vi "QuickSort(Unsigned Byte).vi"(11 "Array In":u8[](array[numeric])) -> (1 "Indices Out":i32[](array[numeric]), 3 "Array Out":u8[](array[numeric]))   [LabVIEW 2015, in "Sorting.lvlib"]
uses:
  Sorting.lvlib
  QSHelper Instances/QSHelper(Unsigned Byte).vi
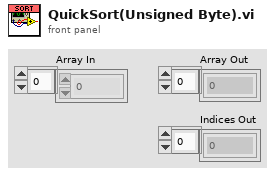
[diagram p1: front panel]
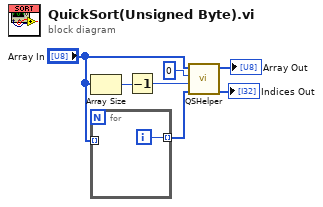
[diagram p0: block diagram]
diagram:
  n1 = Array Size(array="Array In") -> (size(s)=w6:i32)
  n2 = for {
    tunnel: "Array In" -> [_] mode=indexing
    tunnel: [w8] -> w2 mode=indexing
    i -> [w8]
  }
  n3 = Decrement(x=w6) -> (x-1=w5:i32)
  n4 = call-poly "QSHelper.vi"("Indices In"=w2, "hi"=w5, "lo"=0, "Array In"="Array In") -> ("Indices Out"=→"Indices Out":i32[], "Array Out"=→"Array Out":u8[])  [unwired: 6 in]
